vi "tlc_Display Module.vi"(7 "Command (Update UI)":T3=enum."Update UI", 8 "error in (no error)":errorcluster, 9 "Data":variant, 10 "Data Type":T2, 11 "tlc_Display Queue Reference.ctl":T1) -> (0 "error out":errorcluster)   [LabVIEW 2010]
uses:
  tlc_Display_Command Control.ctl
  Controls/tlc_User Interface Data Type.ctl
  Controls/tlc_Display Queue Reference.ctl
  Controls/tlc_User Interface Command.ctl
panel:
  # "Input Data"
  # "Local Data"
  # "Output Data"
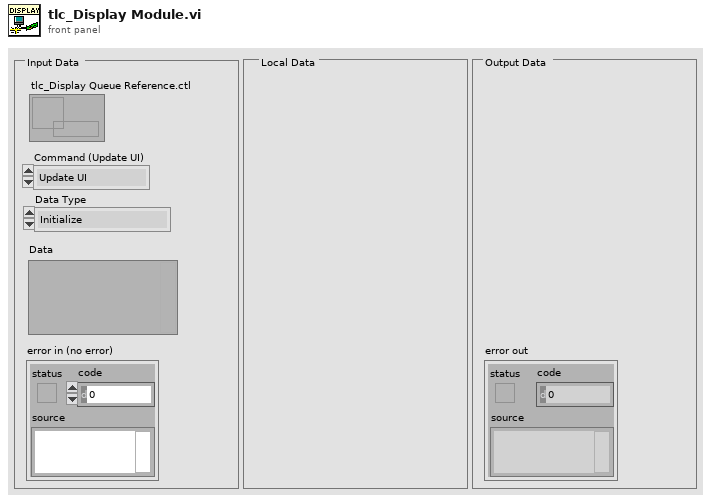
[diagram p1: front panel]
types:
  T1 = typedef "tlc_Display Queue Reference.ctl" = refnum<queue>
  T2 = typedef "tlc_User Interface Data Type.ctl" = enum16{"Initialize", "Initialize Front Panel", "Update Front Panel Channels", "Select Cue in Cue List", "Enable/Disable Front Panel Controls", "Update Cue List", "Stop"}
  T3 = typedef "tlc_Display_Command Control.ctl" = enum16{"Initialize", "Update UI", "Shutdown"}
  T4 = typedef "tlc_User Interface Command.ctl" = cluster{"Data Type":T2, "Data":variant}
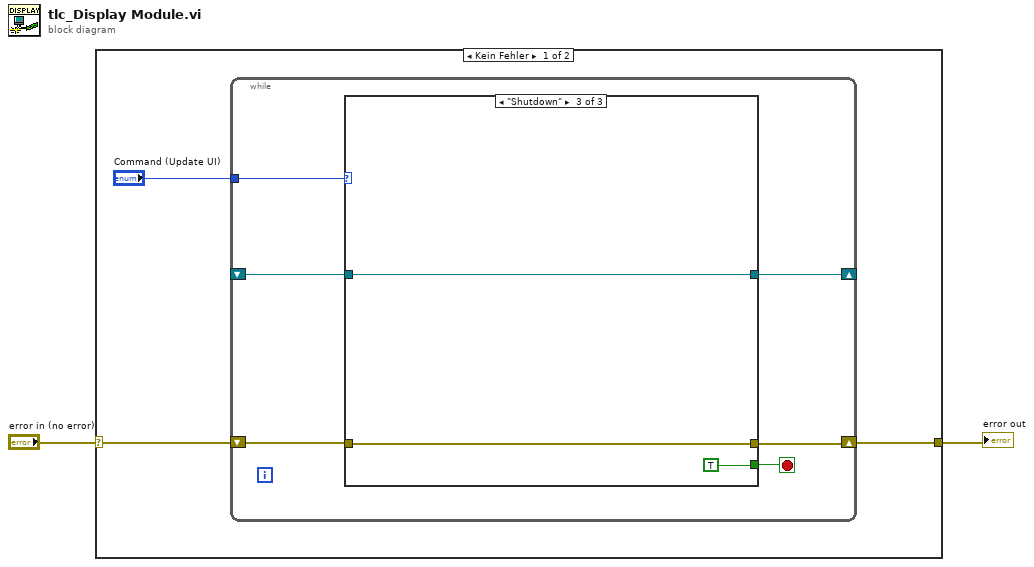
[diagram p0: block diagram]
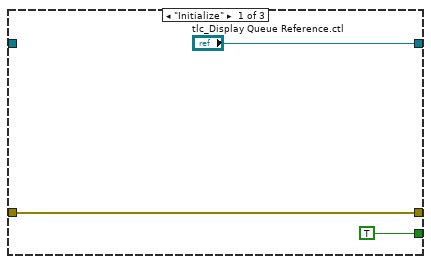
[diagram p2: hidden frame]
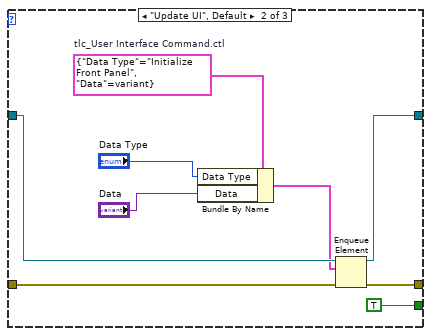
[diagram p3: hidden frame]
diagram:
  n1 = case shown="Kein Fehler" "error in (no error)" {
    selector: "error in (no error)" -> [w5 w27]
    tunnel: [w4 w27] -> w1
    frame No Error {
      n2 = while {
        shift-right: [w9] -> w4
        shift-left: w5 -> [w10]
        tunnel: "Command (Update UI)" -> [w8]
        shift-right: [w7] -> _
        shift-left: _ -> [w6]
        stop <- w11 stop-if-true
        n3 = case shown="\"Shutdown\"" w8 {
          tunnel: [TRUE TRUE TRUE] -> w11
          tunnel: w10 -> [w13 w19 w26]
          tunnel: [w13 w18 w26] -> w9
          tunnel: ["tlc_Display Queue Reference.ctl" w15 w24] -> w7
          tunnel: w6 -> [_ w17 w24]
          frame "Initialize" {
          }
          frame "Update UI", Default {
            w22 = T4 {"Data Type"=enum."Initialize Front Panel", "Data"=variant}  # tlc_User Interface Command.ctl
            n4 = Bundle By Name(cluster=w22, "Data Type"="Data Type", "Data"="Data") -> (w16:T4)
            n5 = Enqueue Element(queue=w17, element=w16, error in (no error)=w19) -> (queue out=w15:T1, error out=w18:errorcluster)  [unwired: 1 in, 1 out]
          }
          frame "Shutdown" {
          }
        }
      }
    }
    frame Error {
    }
  }
  "error out" <- w1
